vi "TDMS Start New File.vi"(8 "error in":errorcluster, 11 "Previous TDMS Refnum In":refnum<k34>) -> (0 "error out":errorcluster, 3 "New TDMS Refnum Out":refnum<k34>)   [LabVIEW 2020]
uses:
  TDMS Global.vi
panel:
  # "Call this when Previous TDMS reaches max size and we need to start a new TDMS file. This VI closes the previous TDMS file and creates a new one with the same settings."
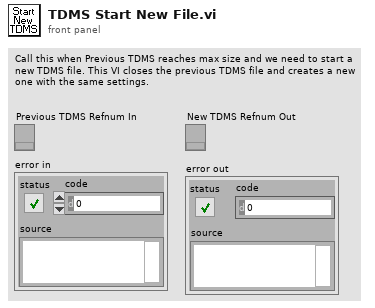
[diagram p1: front panel]
types:
  T1 = typedef "Image Type" = u32
  T2 = enum16{"open", "open or create", "create or replace", "create", "open (read-only)"}
  T3 = enum32{"Bad", "Idle", "Run top level", "Running"}
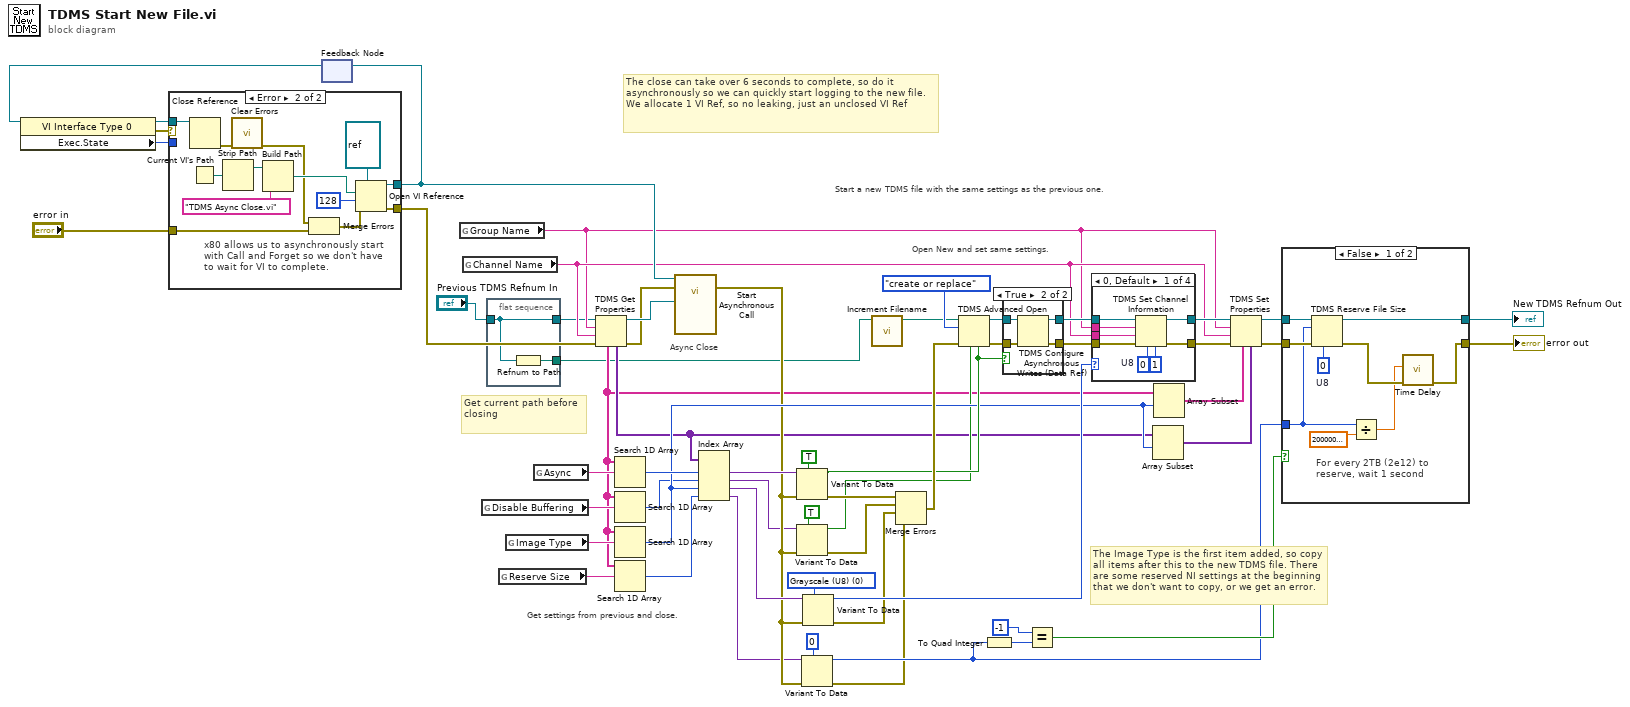
[diagram p0: block diagram]
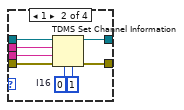
[diagram p4: hidden frame]
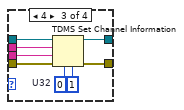
[diagram p5: hidden frame]
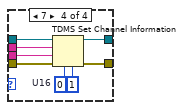
[diagram p6: hidden frame]
diagram:
  w50 = T1 0 items=["Grayscale (U8)", "Grayscale (I16)", "Grayscale (SGL)", "Complex (CSG)", "RGB (U32)", "HSL (U32)", "RGB (U64)", "Grayscale (U16)"] ("Image Type")
  # "Get current path before closing"
  # "The close can take over 6 seconds to complete, so do it asynchronously so we can quickly start logging to the new file. We allocate 1 VI Ref, so no leaking, just an unclosed VI Ref"
  # "The Image Type is the first item added, so copy all items after this to the new TDMS file. There are some reserved NI settings at the beginning that we don't want to copy, or we get an error."
  # "Async Close"
  # "Open New and set same settings."
  # "Get settings from previous and close."
  # "Start a new TDMS file with the same settings as the previous one."
  n1 = feedback #1() -> (w44:refnum<vi>)  [unwired: 1 in]
  n2 = property class="VI Interface Type 0"(reference=w44) -> (reference out=w41:refnum<vi>, error out=w43:errorcluster, "Exec.State"=w42:T3)  [unwired: 1 in]
  n3 = case shown="Error" w43 {
    tunnel: [w61 w72] -> w45
    tunnel: w42 -> [_ _]
    tunnel: w41 -> [w61 w66]
    tunnel: [w60 w71] -> w31
    tunnel: "error in" -> [w60 w64]
    frame No Error {
    }
    frame Error {
      # "x80 allows us to asynchronously start with Call and Forget so we don't have to wait for VI to complete."
      n4 = Close Reference(reference=w66) -> (error out=w65:errorcluster)  [unwired: 1 in]
      n5 = Current VI's Path() -> (path=w68:path)
      n6 = Strip Path(path=w68) -> (stripped path=w69:path)  [unwired: 1 out]
      n7 = call <vilib>:"Clear Errors.vi"("error in (no error)"=w65) -> ("error out"=w62:errorcluster)  [unwired: 5 in, 1 out]
      n8 = Build Path(base path=w69, name or relative path="TDMS Async Close.vi") -> (appended path=w67:path)
      n9 = Merge Errors(w62, w64) -> (w63:errorcluster)
      n10 = Open VI Reference(type specifier VI Refnum (for type only)=refnum<vi> refnum, vi path=w67, options=128, error in (no error)=w63) -> (vi reference=w72:refnum<vi>, error out=w71:errorcluster)  [unwired: 2 in]
    }
  }
  n11 = feedback-in #1(w45) -> ()
  n12 = global read "TDMS Global.vi" "Group Name"() -> (w9:string)
  n13 = global read "TDMS Global.vi" "Channel Name"() -> (w10:string)
  n14 = global read "TDMS Global.vi" "Disable Buffering"() -> (w13:string)
  n15 = flat-sequence {
    tunnel: "Previous TDMS Refnum In" -> [w75]
    tunnel: [w76] -> w3
    tunnel: [w75] -> w2
    frame #0 {
      n16 = Refnum to Path(1:w75) -> (0:w76:path)
    }
  }
  n17 = global read "TDMS Global.vi" "Reserve Size"() -> (w11:string)
  n18 = global read "TDMS Global.vi" "Image Type"() -> (w12:string)
  n19 = global read "TDMS Global.vi" "Async"() -> (w14:string)
  n20 = TDMS Get Properties(8:w31, 9:w10, 10:w9, 11:w2) -> (0:w46:errorcluster, 3:w47:refnum<k34>, 4:w8:variant[], 6:w5:string[])  [unwired: 2 in, 2 out]
  n21 = Search 1D Array(1D array=w5, element=w14) -> (index of element=w56:i32)  [unwired: 1 in]
  n22 = Search 1D Array(1D array=w5, element=w13) -> (index of element=w22:i32)  [unwired: 1 in]
  n23 = Search 1D Array(1D array=w5, element=w12) -> (index of element=w23:i32)  [unwired: 1 in]
  n24 = Search 1D Array(1D array=w5, element=w11) -> (index of element=w7:i32)  [unwired: 1 in]
  n25 = call-by-ref "Start Asynchronous Call"(reference=w45, error in=w46, "tdms file"=w47) -> (error out=w17:errorcluster)  [unwired: 11 in, 1 out]
  n26 = Index Array(array=w8, index #1=w56, index #2=w22, index #3=w23, index #4=w7) -> (element #1=w55:variant, element #2=w16:variant, element #3=w21:variant, element #4=w6:variant)
  n27 = Variant To Data(error in=w17, type=TRUE, Variant=w55) -> (data=w24:bool, error out=w48:errorcluster)
  n28 = Variant To Data(error in=w17, type=TRUE, Variant=w16) -> (data=w15:bool, error out=w19:errorcluster)
  n29 = Variant To Data(error in=w17, type=u64 0, Variant=w6) -> (data=w34:u64, error out=w1:errorcluster)
  n30 = Variant To Data(error in=w17, type=w50, Variant=w21) -> (data=w49:T1, error out=w20:errorcluster)
  n31 = call "Increment Filename.vi"("Path In"=w3) -> ("Incremented Path Out"=w26:path)  [unwired: 10 in]
  n32 = Merge Errors(w48, w19, w20, w1) -> (w27:errorcluster)
  n33 = TDMS Advanced Open(4:w24, 6:w15, 8:w27, 10:T2."create or replace" ("operation (0:open)"), 11:w26) -> (0:w59:errorcluster, 3:w58:refnum<k34>)  [unwired: 1 out]
  n34 = To Quad Integer(1:w34) -> (0:w37:i64)
  n35 = case shown="True" w24 {
    tunnel: [w77 w79] -> w51
    tunnel: w59 -> [w77 w81]
    tunnel: w58 -> [w78 w82]
    tunnel: [w78 w80] -> w52
    frame False {
    }
    frame True {
      n36 = TDMS Configure Asynchronous Writes (Data Ref)(8:w81, 11:w82) -> (0:w79:errorcluster, 3:w80:refnum<k34>)  [unwired: 2 in]
    }
  }
  n37 = Equal?(x=i64 -1, y=w37) -> (x = y?=w35:bool)
  n38 = case shown="0, Default" w49 {
    tunnel: w52 -> [w90 w98 w106 w114]
    tunnel: [w89 w97 w105 w113] -> w53
    tunnel: w51 -> [w88 w96 w104 w112]
    tunnel: [w86 w94 w102 w110] -> w54
    tunnel: w10 -> [w84 w91 w99 w107]
    tunnel: w9 -> [w83 w92 w100 w108]
    frame 0, Default {
      w85 = u8 0  # U8
      n39 = TDMS Set Channel Information(4:u32 1 ("samples per channel"), 6:w85, 8:w88, 9:w84, 10:w83, 11:w90) -> (0:w89:errorcluster, 3:w86:refnum<k34>)  [unwired: 1 in]
    }
    frame 1 {
      w93 = i16 0  # I16
      n40 = TDMS Set Channel Information(4:u32 1 ("samples per channel"), 6:w93, 8:w96, 9:w91, 10:w92, 11:w98) -> (0:w97:errorcluster, 3:w94:refnum<k34>)  [unwired: 1 in]
    }
    frame 4 {
      w101 = u32 0  # U32
      n41 = TDMS Set Channel Information(4:u32 1 ("samples per channel"), 6:w101, 8:w104, 9:w99, 10:w100, 11:w106) -> (0:w105:errorcluster, 3:w102:refnum<k34>)  [unwired: 1 in]
    }
    frame 7 {
      w109 = u16 0  # U16
      n42 = TDMS Set Channel Information(4:u32 1 ("samples per channel"), 6:w109, 8:w112, 9:w107, 10:w108, 11:w114) -> (0:w113:errorcluster, 3:w110:refnum<k34>)  [unwired: 1 in]
    }
  }
  n43 = Array Subset(array=w8, index=w23) -> (w29:variant[])  [unwired: 1 in]
  n44 = Array Subset(array=w5, index=w23) -> (w30:string[])  [unwired: 1 in]
  n45 = TDMS Set Properties(5:w29, 7:w30, 8:w53, 9:w10, 10:w9, 11:w54) -> (0:w28:errorcluster, 3:w39:refnum<k34>)  [unwired: 2 out]
  n46 = case shown="False" w35 {
    tunnel: w28 -> [w121 w124]
    tunnel: w39 -> [w123 w125]
    tunnel: [w122 w125] -> w38
    tunnel: [w118 w124] -> w32
    tunnel: w34 -> [w117 _]
    frame False {
      w120 = u8 0  # U8
      # "For every 2TB (2e12) to reserve, wait 1 second"
      n47 = TDMS Reserve File Size(6:w120, 8:w121, 10:w117, 11:w123) -> (0:w119:errorcluster, 3:w122:refnum<k34>)  [unwired: 1 in]
      n48 = Divide(x=w117, y=2000000000000.0) -> (x/y=w115:dbl)
      n49 = call "Time Delay"("error in (no error)"=w119, "Delay Time (s)"=w115) -> ("error out"=w118:errorcluster)  [unwired: 9 in]
    }
    frame True {
    }
  }
  "error out" <- w32
  "New TDMS Refnum Out" <- w38
